vi "experiment control.vi"() -> ()   [LabVIEW 2012] (continued)
            n1914 = Not(x=w4339) -> (.not. x?=w4338:bool)
            n1915 = Bundle By Name(cluster=w4340, "detected"=w4338) -> (w4333:T26)
            n1916 = local write "Trap DDS"(w4333) -> ()
          }
          frame "Trap DDS: IOUpdate" {
            n1917 = local read "Trap DDS"() -> (w4347:T26)
            n1918 = Unbundle By Name(w4347) -> ("detected"=w4348:bool)
            n1919 = case shown="True" w4348 {
              tunnel: w4347 -> [_ w4358]
              tunnel: w4350 -> [w4352 w4355]
              tunnel: [w4352 w4353] -> w4349
              frame False {
              }
              frame True {
                n1920 = Unbundle By Name(w4358) -> ("usb 1"=w4357:refnum<visa-resource-name>, "usb 2"=w4356:refnum<visa-resource-name>)
                n1921 = call "DDS9959 IO Update.vi"("error in (no error)"=w4355, "VISA resource name"=w4357) -> ("error out"=w4354:errorcluster)  [unwired: 4 in, 1 out]
                n1922 = call "DDS9959 IO Update.vi"("error in (no error)"=w4354, "VISA resource name"=w4356) -> ("error out"=w4353:errorcluster)  [unwired: 4 in, 1 out]
              }
            }
          }
          frame "Trap DDS: Upload" {
            n1923 = local read "Trap DDS"() -> (w4360:T26)
            n1924 = Unbundle By Name(w4360) -> ("detected"=w4361:bool)
            n1925 = case shown="True" w4361 {
              tunnel: w4360 -> [_ w4372]
              tunnel: w4363 -> [w4365 w4370]
              tunnel: [w4365 w4371] -> w4362
              frame False {
              }
              frame True {
                n1926 = Unbundle By Name(w4372) -> ("load ARR"=w4369:bool, "ramp enable"=w4368:bool, "channels"=w4373:T95, "Global\nScale Factor"=w4367:dbl, "ramp time"=w4366:u8)
                n1927 = Unbundle By Name(w4372) -> ("usb 1"=w4380:refnum<visa-resource-name>, "clock"=w4382:dbl, "pll multiplier"=w4383:u8, "usb 2"=w4381:refnum<visa-resource-name>)
                n1928 = Array Subset(array=w4373, index=0, length=4) -> (w4378:T95)
                n1929 = Array Subset(array=w4373, index=4, length=4) -> (w4379:T95)
                n1930 = Multiply(x=w4382, y=w4383) -> (x*y=w4384:dbl)
                n1931 = for {
                  tunnel: w4378 -> [w4430] mode=indexing
                  tunnel: w4379 -> [w4429] mode=indexing
                  tunnel: w4380 -> [w4428]
                  tunnel: w4381 -> [w4423]
                  tunnel: w4384 -> [w4420]
                  shift-right: [w4396] -> w4371
                  shift-left: w4370 -> [w4395]
                  tunnel: w4369 -> [w4393]
                  tunnel: w4368 -> [w4392]
                  tunnel: w4366 -> [w4391]
                  tunnel: w4367 -> [w4386]
                  i -> [w4419]
                  w4385 = "04" ("Register")
                  n1932 = Unbundle By Name(w4430) -> ("Frequency"=w4401:dbl, "Phase"=w4422:dbl, "Amplitude"=w4390:dbl)
                  n1933 = Unbundle By Name(w4429) -> ("Frequency"=w4399:dbl, "Phase"=w4421:dbl, "Amplitude"=w4388:dbl)
                  n1934 = Increment(x=w4419) -> (x+1=w4414:i32)
                  n1935 = expression code="x/1000"(w4401) -> (w4400:dbl)
                  n1936 = expression code="x/1000"(w4399) -> (w4398:dbl)
                  n1937 = Bundle By Name(cluster=T48 {"load ARR at ioupdate"=FALSE, "ramp enable"=FALSE, "amplitude multiplier enable"=FALSE, "open"=FALSE, "inc/dec step size (14)"=FALSE, "inc/dec step size (15)"=FALSE} ("Amplitude Control Register"), "load ARR at ioupdate"=w4393, "ramp enable"=w4392, "amplitude multiplier enable"=TRUE) -> (w4413:T48)
                  n1938 = call "DDS9959 Set Frequency.vi"("VISA resource name"=w4428, "Register"=w4385, "Set Frequency (MHz)"=w4400, "Channel"=w4414, "Clock Frequency (MHz)"=w4420, "error in (no error)"=w4395) -> ("VISA resource name out"=w4427:refnum<visa-resource-name>, "error out"=w4404:errorcluster)  [unwired: 8 in]
                  n1939 = call "DDS9959 Set Phase.vi"("VISA resource name"=w4427, "Set Phase (Deg)"=w4422, "Channel"=w4414, "error in (no error)"=w4404) -> ("VISA resource name out"=w4426:refnum<visa-resource-name>, "error out"=w4405:errorcluster)  [unwired: 10 in]
                  n1940 = Multiply(x=w4386, y=w4390) -> (x*y=w4389:dbl)
                  n1941 = Multiply(x=w4386, y=w4388) -> (x*y=w4387:dbl)
                  n1942 = call "DDS9959 Set Amplitude.vi"("VISA resource name"=w4426, "ramp rate"=w4391, "Set Amplitude Scale Factor"=w4389, "Channel"=w4414, "Amplitude Control Register"=w4413, "error in (no error)"=w4405) -> ("VISA resource name out"=w4417:refnum<visa-resource-name>, "error out"=w4418:errorcluster)  [unwired: 8 in]
                  n1943 = Bundle By Name(cluster=T49 {"0=cos, 1=sin"=FALSE, "clear phase accum"=FALSE, "autoclear phase accum"=FALSE, "clear sweep accum"=FALSE, "autoclear sweep accum"=FALSE, "match pipe delays"=FALSE, "DAC power down"=FALSE, "digital power down"=FALSE, "DAC current (8)"=FALSE, "DAC current (9)"=FALSE, "Must be 0"=FALSE, "Open"=FALSE, "Open"=FALSE, "Sweep ramp rate timer"=FALSE, "Sweep enable"=FALSE, "Sweep no-dwell"=FALSE, "Open"=FALSE, "Open"=FALSE, "Open"=FALSE, "Open"=FALSE, "Open"=FALSE, "Open 2"=FALSE, "AFP mod select (22)"=FALSE, "AFP mod select (23)"=FALSE} ("Channel Function Register"), "clear phase accum"=FALSE, "autoclear phase accum"=FALSE, "DAC current (8)"=TRUE, "DAC current (9)"=TRUE) -> (w4407:T49)
                  n1944 = call "DDS9959 Set CFR.vi"("error in (no error)"=w4418, "Channel"=w4414, "Channel Function Register"=w4407, "VISA resource name"=w4417) -> ("error out"=w4397:errorcluster)  [unwired: 1 out]
                  n1945 = call "DDS9959 Set Frequency.vi"("VISA resource name"=w4423, "Register"=w4385, "Set Frequency (MHz)"=w4398, "Channel"=w4414, "Clock Frequency (MHz)"=w4420, "error in (no error)"=w4397) -> ("VISA resource name out"=w4425:refnum<visa-resource-name>, "error out"=w4403:errorcluster)  [unwired: 8 in]
                  n1946 = call "DDS9959 Set Phase.vi"("VISA resource name"=w4425, "Set Phase (Deg)"=w4421, "Channel"=w4414, "error in (no error)"=w4403) -> ("VISA resource name out"=w4424:refnum<visa-resource-name>, "error out"=w4402:errorcluster)  [unwired: 10 in]
                  n1947 = call "DDS9959 Set Amplitude.vi"("VISA resource name"=w4424, "ramp rate"=w4391, "Set Amplitude Scale Factor"=w4387, "Channel"=w4414, "Amplitude Control Register"=w4413, "error in (no error)"=w4402) -> ("VISA resource name out"=w4416:refnum<visa-resource-name>, "error out"=w4415:errorcluster)  [unwired: 8 in]
                  n1948 = call "DDS9959 Set CFR.vi"("error in (no error)"=w4415, "Channel"=w4414, "Channel Function Register"=w4407, "VISA resource name"=w4416) -> ("error out"=w4396:errorcluster)  [unwired: 1 out]
                }
              }
            }
          }
          frame "Trap DDS: Upload Ramp" {
            n1949 = local read "Trap DDS"() -> (w4433:T26)
            n1950 = Unbundle By Name(w4433) -> ("ramp"=w4432:T113, "232"=w4431:refnum<visa-resource-name>)
            n1951 = for {
              tunnel: w4432 -> [w4486] mode=indexing
              shift-right: [w4439] -> w4435
              shift-left: w4436 -> [w4464]
              shift-right: [w4440] -> _
              shift-left: w4431 -> [w4463]
              i -> [w4455]
              w4450 = i16 0 ("lower limit")
              w4449 = i16 1023 ("upper limit")
              w4444 = "w" ("string")
              n1952 = Unbundle By Name(w4486) -> ("start"=w4485:dbl, "end"=w4484:dbl, "ramp time"=w4472:u8, "edge"=w4442:bool)
              n1953 = expression code="x*1024"(w4485) -> (w4483:dbl)
              n1954 = expression code="x*1024"(w4484) -> (w4482:dbl)
              n1955 = Number To Decimal String(number=w4455) -> (decimal integer string=w4443:string)  [unwired: 1 in]
              n1956 = To Word Integer(number=w4483) -> (16bit integer=w4459:i16)
              n1957 = To Word Integer(number=w4482) -> (16bit integer=w4456:i16)
              n1958 = Subtract(x=w4459, y=w4456) -> (x-y=w4479:i16)
              n1959 = Absolute Value(x=w4479) -> (abs(x)=w4478:i16)
              n1960 = Divide(x=w4478, y=i16 1024) -> (x/y=w4476:dbl)
              n1961 = Divide(x=u8 185, y=w4472) -> (x/y=w4470:dbl)
              n1962 = Multiply(x=w4476, y=w4470) -> (x*y=w4475:dbl)
              n1963 = To Unsigned Byte Integer(number=w4475) -> (unsigned 8bit integer=w4454:u8)
              n1964 = case shown="True" w4442 {
                tunnel: ["r" "f"] -> w4441
                frame True {
                }
                frame False {
                }
              }
              n1965 = In Range and Coerce(upper limit=w4449, x=w4459, lower limit=w4450) -> (coerced(x)=w4458:i16)  [unwired: 1 out]
              n1966 = In Range and Coerce(upper limit=w4449, x=w4456, lower limit=w4450) -> (coerced(x)=w4457:i16)  [unwired: 1 out]
              n1967 = In Range and Coerce(upper limit=u8 255, x=w4454, lower limit=u8 1) -> (coerced(x)=w4453:u8)  [unwired: 1 out]
              n1968 = Type Cast(x=w4458) -> (*(type *) &x=w4481:string)  [unwired: 1 in]
              n1969 = Type Cast(x=w4457) -> (*(type *) &x=w4480:string)  [unwired: 1 in]
              n1970 = Type Cast(x=w4453) -> (*(type *) &x=w4474:string)  [unwired: 1 in]
              n1971 = Concatenate Strings(w4444, w4443, "b" ("string"), w4481) -> (w4462:string)
              n1972 = Concatenate Strings(w4444, w4443, "e" ("string"), w4480) -> (w4467:string)
              n1973 = Concatenate Strings(w4444, w4443, "s" ("string"), w4474) -> (w4446:string)
              n1974 = Concatenate Strings(w4444, w4443, w4441) -> (w4445:string)
              n1975 = VISA Write(VISA resource name=w4463, write buffer=w4462, error in (no error)=w4464) -> (VISA resource name out=w4468:refnum<visa-resource-name>, error out=w4469:errorcluster)  [unwired: 1 out]
              n1976 = VISA Write(VISA resource name=w4468, write buffer=w4467, error in (no error)=w4469) -> (VISA resource name out=w4465:refnum<visa-resource-name>, error out=w4466:errorcluster)  [unwired: 1 out]
              n1977 = VISA Write(VISA resource name=w4465, write buffer=w4446, error in (no error)=w4466) -> (VISA resource name out=w4448:refnum<visa-resource-name>, error out=w4447:errorcluster)  [unwired: 1 out]
              n1978 = Wait (ms)(milliseconds to wait=u32 50) -> ()  [unwired: 1 out]
              n1979 = VISA Write(VISA resource name=w4448, write buffer=w4445, error in (no error)=w4447) -> (VISA resource name out=w4440:refnum<visa-resource-name>, error out=w4439:errorcluster)  [unwired: 1 out]
            }
          }
          frame "Trap DDS: Connect Serial" {
            n1980 = local read "Trap DDS"() -> (w4490:T26)
            n1981 = Unbundle By Name(w4490) -> ("232"=w4489:refnum<visa-resource-name>)
            n1982 = call-poly "VISA Configure Serial Port"("VISA resource name"=w4489, "Enable Termination\nChar (T)"=FALSE ("Enable Termination\nChar (T)"), "error in (no error)"=w4494) -> ("error out"=w4493:errorcluster)  [unwired: 11 in, 1 out]
          }
          frame "Trap DDS: Disconnect Serial" {
            n1983 = local read "Trap DDS"() -> (w4497:T26)
            n1984 = Unbundle By Name(w4497) -> ("232"=w4496:refnum<visa-resource-name>)
            n1985 = VISA Close(VISA resource name=w4496, error in (no error)=w4500) -> (error out=w4499:errorcluster)
          }
          frame "Trap DDS: Zero" {
            n1986 = local read "Trap DDS"() -> (w4504:T26)
            n1987 = Unbundle By Name(w4504) -> ("detected"=w4505:bool)
            n1988 = case shown="True" w4505 {
              tunnel: w4504 -> [_ w4514]
              tunnel: w4507 -> [w4509 w4512]
              tunnel: [w4509 w4513] -> w4506
              tunnel: [_ "Trap DDS: IOUpdate" ("State(s) in (\"\")")] -> w4502
              frame False {
              }
              frame True {
                n1989 = Unbundle By Name(w4514) -> ("usb 1"=w4515:refnum<visa-resource-name>, "usb 2"=w4516:refnum<visa-resource-name>)
                n1990 = for {
                  N: 4 -> [_]
                  tunnel: w4515 -> [w4520]
                  tunnel: w4516 -> [w4518]
                  shift-right: [w4521] -> w4513
                  shift-left: w4512 -> [w4519]
                  i -> [w4527]
                  n1991 = Increment(x=w4527) -> (x+1=w4526:i32)
                  n1992 = Bundle By Name(cluster=T49 {"0=cos, 1=sin"=FALSE, "clear phase accum"=FALSE, "autoclear phase accum"=FALSE, "clear sweep accum"=FALSE, "autoclear sweep accum"=FALSE, "match pipe delays"=FALSE, "DAC power down"=FALSE, "digital power down"=FALSE, "DAC current (8)"=FALSE, "DAC current (9)"=FALSE, "Must be 0"=FALSE, "Open"=FALSE, "Open"=FALSE, "Sweep ramp rate timer"=FALSE, "Sweep enable"=FALSE, "Sweep no-dwell"=FALSE, "Open"=FALSE, "Open"=FALSE, "Open"=FALSE, "Open"=FALSE, "Open"=FALSE, "Open 2"=FALSE, "AFP mod select (22)"=FALSE, "AFP mod select (23)"=FALSE} ("Channel Function Register"), "clear phase accum"=TRUE, "autoclear phase accum"=FALSE) -> (w4523:T49)
                  n1993 = call "DDS9959 Set CFR.vi"("error in (no error)"=w4519, "Channel"=w4526, "Channel Function Register"=w4523, "VISA resource name"=w4520) -> ("error out"=w4517:errorcluster)  [unwired: 1 out]
                  n1994 = call "DDS9959 Set CFR.vi"("error in (no error)"=w4517, "Channel"=w4526, "Channel Function Register"=w4523, "VISA resource name"=w4518) -> ("error out"=w4521:errorcluster)  [unwired: 1 out]
                }
              }
            }
            n1995 = Enqueue Element At Opposite End(queue=w4503, element=w4502) -> ()  [unwired: 2 in, 3 out]
          }
          frame "Trap DDS: Reset" {
            n1996 = local read "Trap DDS"() -> (w4528:T26)
            n1997 = Unbundle By Name(w4528) -> ("detected"=w4529:bool)
            n1998 = case shown="True" w4529 {
              tunnel: w4528 -> [_ w4553]
              tunnel: w4532 -> [w4534 w4541]
              tunnel: [w4534 w4539] -> w4531
              frame False {
              }
              frame True {
                w4549 = T104 {"system clock offset"=FALSE, "system clock offset"=FALSE, "open"=FALSE, "open"=FALSE, "multidevice sync mask"=FALSE, "multidevice sync status"=FALSE, "sync master enable"=FALSE, "auto sync enable"=FALSE, "open"=FALSE, "open"=FALSE, "open"=FALSE, "open"=FALSE, "all channel clear phase accumulator"=FALSE, "all channel autoclear phase accumulator"=FALSE, "all channel clear sweep accumulator"=FALSE, "all channel autoclear sweep accumulator"=FALSE} ("Channel Function Register")
                n1999 = Unbundle By Name(w4553) -> ("usb 1"=w4552:refnum<visa-resource-name>, "usb 2"=w4542:refnum<visa-resource-name>)
                n2000 = Bundle By Name(cluster=w4549, "all channel clear phase accumulator"=TRUE) -> (w4547:T104)
                n2001 = call "DDS9959 Set FR2.vi"("error in (no error)"=w4541, "Channel Function Register"=w4547, "VISA resource name"=w4552) -> ("error out"=w4540:errorcluster, "VISA resource name out"=w4546:refnum<visa-resource-name>)  [unwired: 3 in]
                n2002 = Bundle By Name(cluster=w4549, "all channel clear phase accumulator"=FALSE) -> (w4548:T104)
                n2003 = call "DDS9959 IO Update.vi"("error in (no error)"=w4540, "VISA resource name"=w4546) -> ("error out"=w4536:errorcluster, "VISA resource name out"=w4545:refnum<visa-resource-name>)  [unwired: 4 in]
                n2004 = call "DDS9959 Set FR2.vi"("error in (no error)"=w4536, "Channel Function Register"=w4548, "VISA resource name"=w4545) -> ("error out"=w4535:errorcluster)  [unwired: 3 in, 1 out]
                n2005 = call "DDS9959 Set FR2.vi"("error in (no error)"=w4535, "Channel Function Register"=w4547, "VISA resource name"=w4542) -> ("error out"=w4537:errorcluster, "VISA resource name out"=w4544:refnum<visa-resource-name>)  [unwired: 3 in]
                n2006 = call "DDS9959 IO Update.vi"("error in (no error)"=w4537, "VISA resource name"=w4544) -> ("error out"=w4538:errorcluster, "VISA resource name out"=w4543:refnum<visa-resource-name>)  [unwired: 4 in]
                n2007 = call "DDS9959 Set FR2.vi"("error in (no error)"=w4538, "Channel Function Register"=w4548, "VISA resource name"=w4543) -> ("error out"=w4539:errorcluster)  [unwired: 3 in, 1 out]
              }
            }
          }
          frame "---------- Trap DDS ----------" {
            # "Template Separator\n(You can make a copy of, or modify, this frame)"
          }
          frame "DDS: Set Clock" {
            n2008 = local read "DDS"() -> (w4560:T25)
            n2009 = Unbundle By Name(w4560) -> ("address"=w4564:refnum<visa-resource-name>, "pll multiplier"=w4563:u8, "vco gain"=w4559:bool)
            n2010 = call "DDS9959 Set Clock.vi"("error in (no error)"=w4567, "VCO Gain"=w4559, "PLL Multiplier"=w4563, "VISA resource name"=w4564) -> ("error out"=w4566:errorcluster, "VISA resource name out"=w4561:refnum<visa-resource-name>)  [unwired: 6 in]
            n2011 = Unbundle By Name(w4566) -> ("status"=w4558:bool)
            n2012 = Not(x=w4558) -> (.not. x?=w4557:bool)
            n2013 = Bundle By Name(cluster=w4560, "address"=w4561, "detected"=w4557) -> (w4562:T25)
            n2014 = local write "DDS"(w4562) -> ()
          }
          frame "DDS: Set Frequency Ramp" {
            n2015 = local read "DDS"() -> (w4569:T25)
            n2016 = Unbundle By Name(w4569) -> ("address"=w4573:refnum<visa-resource-name>, "frequency ramp"=w4574:bool, "clock"=w4572:dbl)
            n2017 = case shown="True" w4574 {
              tunnel: w4573 -> [w4579 w4589]
              tunnel: [w4580 w4587] -> w4577
              tunnel: w4576 -> [w4580 w4585]
              tunnel: w4572 -> [_ w4583]
              tunnel: [w4579 w4581] -> w4571
              frame False {
              }
              frame True {
                w4582 = 0.002  # Set Frequency (MHz)
                w4584 = u16 2 ("Channel")
                w4594 = 0.5  # Falling Ramp Step (us)
                n2018 = Bundle By Name(cluster=T49 {"0=cos, 1=sin"=FALSE, "clear phase accum"=FALSE, "autoclear phase accum"=FALSE, "clear sweep accum"=FALSE, "autoclear sweep accum"=FALSE, "match pipe delays"=FALSE, "DAC power down"=FALSE, "digital power down"=FALSE, "DAC current (8)"=TRUE, "DAC current (9)"=TRUE, "Must be 0"=FALSE, "Open"=FALSE, "Open"=FALSE, "Sweep ramp rate timer"=FALSE, "Sweep enable"=FALSE, "Sweep no-dwell"=FALSE, "Open"=FALSE, "Open"=FALSE, "Open"=FALSE, "Open"=FALSE, "Open"=FALSE, "Open 2"=FALSE, "AFP mod select (22)"=FALSE, "AFP mod select (23)"=FALSE} ("Channel Function Register"), "Sweep enable"=TRUE, "Sweep no-dwell"=FALSE, "AFP mod select (22)"=FALSE, "AFP mod select (23)"=TRUE) -> (w4601:T49)
                n2019 = call "DDS9959 Set CFR.vi"("error in (no error)"=w4585, "Channel"=w4584, "Channel Function Register"=w4601, "VISA resource name"=w4589) -> ("error out"=w4590:errorcluster, "VISA resource name out"=w4591:refnum<visa-resource-name>)
                n2020 = call "DDS9959 Set Frequency.vi"("VISA resource name"=w4591, "Register"="08", "Set Frequency (MHz)"=w4582, "Channel"=w4584, "Clock Frequency (MHz)"=w4583, "error in (no error)"=w4590) -> ("VISA resource name out"=w4592:refnum<visa-resource-name>, "error out"=w4586:errorcluster)  [unwired: 8 in]
                n2021 = call "DDS9959 Set Frequency.vi"("VISA resource name"=w4592, "Register"="08", "Set Frequency (MHz)"=w4582, "Channel"=w4584, "Clock Frequency (MHz)"=w4583, "error in (no error)"=w4586) -> ("VISA resource name out"=w4593:refnum<visa-resource-name>, "error out"=w4588:errorcluster)  [unwired: 8 in]
                n2022 = call "DDS9959 Set Ramp Rate.vi"("VISA resource name"=w4593, "Falling Ramp Step (us)"=w4594, "Rising Ramp Step (us)"=w4594, "Channel"=w4584, "error in (no error)"=w4588, "Clock Frequency (MHz)"=w4583) -> ("VISA resource name out"=w4581:refnum<visa-resource-name>, "error out"=w4587:errorcluster)  [unwired: 8 in]
              }
            }
            n2023 = Bundle By Name(cluster=w4569, "address"=w4571) -> (w4570:T25)
            n2024 = local write "DDS"(w4570) -> ()
          }
          frame "DDS: Set Frequency" {
            n2025 = local read "DDS"() -> (w4612:T25)
            n2026 = case shown="\"1\", Default" w4618 {
              tunnel: w4612 -> [w4630 w4641 w4652 w4663]
              tunnel: [w4629 w4640 w4651 w4662] -> w4614
              tunnel: [w4624 w4635 w4646 w4657] -> w4605
              tunnel: [w4622 w4633 w4644 w4655] -> w4606
              tunnel: [u16 1 ("Channel") u16 2 ("Channel") u16 3 ("Channel") u16 4 ("Channel")] -> w4604
              tunnel: [w4620 w4631 w4642 w4653] -> w4603
              frame "1", Default {
                n2027 = Unbundle By Name(w4630) -> ("address"=w4629:refnum<visa-resource-name>, "channel 1"=w4623:dbl, "clock"=w4627:dbl, "pll multiplier"=w4626:u8, "channel 1 endramp"=w4621:dbl)
                n2028 = Multiply(x=w4627, y=w4626) -> (x*y=w4625:dbl)
                n2029 = To Double Precision Float(number=w4625) -> (double precision float=w4624:dbl)
                n2030 = expression code="x/2"(w4623) -> (w4622:dbl)
                n2031 = expression code="x/2"(w4621) -> (w4620:dbl)
              }
              frame "2" {
                n2032 = Unbundle By Name(w4641) -> ("address"=w4640:refnum<visa-resource-name>, "channel 2"=w4634:dbl, "clock"=w4638:dbl, "pll multiplier"=w4637:u8, "channel 2 endramp"=w4632:dbl)
                n2033 = Multiply(x=w4638, y=w4637) -> (x*y=w4636:dbl)
                n2034 = To Double Precision Float(number=w4636) -> (double precision float=w4635:dbl)
                n2035 = expression code="x/2"(w4634) -> (w4633:dbl)
                n2036 = expression code="x/2"(w4632) -> (w4631:dbl)
              }
              frame "3" {
                n2037 = Unbundle By Name(w4652) -> ("address"=w4651:refnum<visa-resource-name>, "channel 3"=w4645:dbl, "clock"=w4649:dbl, "pll multiplier"=w4648:u8, "channel 3 endramp"=w4643:dbl)
                n2038 = Multiply(x=w4649, y=w4648) -> (x*y=w4647:dbl)
                n2039 = To Double Precision Float(number=w4647) -> (double precision float=w4646:dbl)
                n2040 = expression code="x/2"(w4645) -> (w4644:dbl)
                n2041 = expression code="x/2"(w4643) -> (w4642:dbl)
              }
              frame "4" {
                n2042 = Unbundle By Name(w4663) -> ("address"=w4662:refnum<visa-resource-name>, "channel 4"=w4656:dbl, "clock"=w4660:dbl, "pll multiplier"=w4659:u8, "channel 4 endramp"=w4654:dbl)
                n2043 = Multiply(x=w4660, y=w4659) -> (x*y=w4658:dbl)
                n2044 = To Double Precision Float(number=w4658) -> (double precision float=w4657:dbl)
                n2045 = expression code="x/2"(w4656) -> (w4655:dbl)
                n2046 = expression code="x/2"(w4654) -> (w4653:dbl)
              }
            }
            n2047 = call "DDS9959 Set Frequency.vi"("VISA resource name"=w4614, "Register"="04", "Set Frequency (MHz)"=w4606, "Channel"=w4604, "Clock Frequency (MHz)"=w4605, "error in (no error)"=w4617) -> ("VISA resource name out"=w4610:refnum<visa-resource-name>, "error out"=w4608:errorcluster)  [unwired: 8 in]
            n2048 = call "DDS9959 Set Frequency.vi"("VISA resource name"=w4610, "Register"="0A", "Set Frequency (MHz)"=w4603, "Channel"=w4604, "Clock Frequency (MHz)"=w4605, "error in (no error)"=w4608) -> ("VISA resource name out"=w4609:refnum<visa-resource-name>, "error out"=w4616:errorcluster)  [unwired: 8 in]
            n2049 = Bundle By Name(cluster=w4612, "address"=w4609) -> (w4613:T25)
            n2050 = local write "DDS"(w4613) -> ()
          }
          frame "DDS: Goto Frequency" {
            n2051 = Match Pattern(string=w4684, regular expression=",") -> (before substring=w4667:string, after substring=w4676:string)  [unwired: 1 in, 2 out]
            n2052 = local read "DDS"() -> (w4669:T25)
            n2053 = case shown="\"1\", Default" w4667 {
              tunnel: w4669 -> [w4730 w4738 w4746 w4754]
              tunnel: [w4729 w4737 w4745 w4753] -> w4681
              tunnel: [w4723 w4731 w4739 w4747] -> w4680
              tunnel: [w4728 w4736 w4744 w4752] -> w4678
              tunnel: [u16 1 ("Channel") u16 2 ("Channel") u16 3 ("Channel") u16 4 ("Channel")] -> w4679
              frame "1", Default {
                n2054 = Unbundle By Name(w4730) -> ("address"=w4729:refnum<visa-resource-name>, "channel 1"=w4728:dbl, "clock"=w4726:dbl, "pll multiplier"=w4725:u8)
                n2055 = Multiply(x=w4726, y=w4725) -> (x*y=w4724:dbl)
                n2056 = To Double Precision Float(number=w4724) -> (double precision float=w4723:dbl)
              }
              frame "2" {
                n2057 = Unbundle By Name(w4738) -> ("address"=w4737:refnum<visa-resource-name>, "channel 2"=w4736:dbl, "clock"=w4734:dbl, "pll multiplier"=w4733:u8)
                n2058 = Multiply(x=w4734, y=w4733) -> (x*y=w4732:dbl)
                n2059 = To Double Precision Float(number=w4732) -> (double precision float=w4731:dbl)
              }
              frame "3" {
                n2060 = Unbundle By Name(w4746) -> ("address"=w4745:refnum<visa-resource-name>, "channel 3"=w4744:dbl, "clock"=w4742:dbl, "pll multiplier"=w4741:u8)
                n2061 = Multiply(x=w4742, y=w4741) -> (x*y=w4740:dbl)
                n2062 = To Double Precision Float(number=w4740) -> (double precision float=w4739:dbl)
              }
              frame "4" {
                n2063 = Unbundle By Name(w4754) -> ("address"=w4753:refnum<visa-resource-name>, "channel 4"=w4752:dbl, "clock"=w4750:dbl, "pll multiplier"=w4749:u8)
                n2064 = Multiply(x=w4750, y=w4749) -> (x*y=w4748:dbl)
                n2065 = To Double Precision Float(number=w4748) -> (double precision float=w4747:dbl)
              }
            }
            n2066 = Fract/Exp String To Number(string=w4676) -> (number=w4672:dbl)  [unwired: 3 in, 1 out]
            n2067 = expression code="x/2"(w4672) -> (w4671:dbl)
            n2068 = expression code="x/2"(w4678) -> (w4673:dbl)
            n2069 = Subtract(x=w4671, y=w4673) -> (x-y=w4675:dbl)
            n2070 = Sign(1:w4675) -> (0:w4674:dbl)
            n2071 = while {
              tunnel: w4680 -> [w4720]
              tunnel: w4679 -> [w4719]
              shift-right: [w4704] -> w4666
              shift-left: w4673 -> [w4705]
              shift-right: [w4706] -> w4682
              shift-left: w4683 -> [w4722]
              tunnel: w4674 -> [w4716]
              tunnel: w4671 -> [w4711]
              tunnel: w4673 -> [w4712]
              shift-right: [w4708] -> w4668
              shift-left: w4681 -> [w4721]
              stop <- w4710 stop-if-true
              n2072 = Multiply(x=w4716, y=0.5) -> (x*y=w4718:dbl)
              n2073 = Wait (ms)(milliseconds to wait=u32 10) -> ()  [unwired: 1 out]
              n2074 = Add(x=w4705, y=w4718) -> (x+y=w4715:dbl)
              n2075 = Max & Min(x=w4712, y=w4711) -> (max(x,y)=w4714:dbl, min(x,y)=w4713:dbl)
              n2076 = In Range and Coerce(upper limit=w4714, x=w4715, lower limit=w4713) -> (coerced(x)=w4704:dbl)  [unwired: 1 out]
              n2077 = Equal?(x=w4704, y=w4711) -> (x = y?=w4710:bool)
              n2078 = call "DDS9959 Set Frequency.vi"("VISA resource name"=w4721, "Register"="04", "Set Frequency (MHz)"=w4704, "Channel"=w4719, "Clock Frequency (MHz)"=w4720, "error in (no error)"=w4722) -> ("VISA resource name out"=w4709:refnum<visa-resource-name>, "error out"=w4707:errorcluster)  [unwired: 8 in]
              n2079 = call "DDS9959 IO Update.vi"("error in (no error)"=w4707, "VISA resource name"=w4709) -> ("error out"=w4706:errorcluster, "VISA resource name out"=w4708:refnum<visa-resource-name>)  [unwired: 4 in]
            }
            n2080 = expression code="2*x"(w4666) -> (w4665:dbl)
            n2081 = case shown="\"1\", Default" w4667 {
              tunnel: [w4689 w4693 w4697 w4701] -> w4670
              tunnel: w4669 -> [w4688 w4692 w4696 w4700]
              tunnel: w4668 -> [w4687 w4691 w4695 w4699]
              tunnel: w4665 -> [w4686 w4690 w4694 w4698]
              frame "1", Default {
                n2082 = Bundle By Name(cluster=w4688, "address"=w4687, "channel 1"=w4686) -> (w4689:T25)
              }
              frame "2" {
                n2083 = Bundle By Name(cluster=w4692, "address"=w4691, "channel 2"=w4690) -> (w4693:T25)
              }
              frame "3" {
                n2084 = Bundle By Name(cluster=w4696, "address"=w4695, "channel 3"=w4694) -> (w4697:T25)
              }
              frame "4" {
                n2085 = Bundle By Name(cluster=w4700, "address"=w4699, "channel 4"=w4698) -> (w4701:T25)
              }
            }
            n2086 = local write "DDS"(w4670) -> ()
          }
          frame "---------- Coils ----------" {
            # "Template Separator\n(You can make a copy of, or modify, this frame)"
          }
          frame "Coils: Initialize" {
            # "Template Separator\n(You can make a copy of, or modify, this frame)"
            n2087 = local read "Coils"() -> (w4762:T15)
            n2088 = Unbundle By Name(w4762) -> ("Keithley USB"=w4768:refnum<visa-resource-name>, "AO Channels"=w4767:tag, "DO Lines"=w4766:tag)
            n2089 = call "CoilsInit.vi"("error in"=w4765, "DO Lines"=w4766, "AO Channels"=w4767, "Keithley USB"=w4768) -> ("error out"=w4759:errorcluster, "DO Task out"=w4763:refnum<k21>, "AO Task out"=w4764:refnum<k21>)  [unwired: 4 in, 1 out]
            n2090 = local write "Coils AO Task:skip"(w4764) -> ()
            n2091 = local write "Coils DO Task:skip"(w4763) -> ()
            n2092 = Unbundle By Name(w4759) -> ("status"=w4758:bool)
            n2093 = case shown="False" w4758 {
              tunnel: w4761 -> [w4772 w4773]
              tunnel: [w4771 w4773] -> w4760
              frame False {
                n2094 = Enqueue Element At Opposite End(queue=w4772, element="Coils: Set") -> (queue out=w4771:refnum<queue>)  [unwired: 2 in, 2 out]
              }
              frame True {
              }
            }
          }
          frame "Coils: Close" {
            # "Template Separator\n(You can make a copy of, or modify, this frame)"
            n2095 = local read "Coils AO Task:skip"() -> (w4775:refnum<k21>)
            n2096 = local read "Coils DO Task:skip"() -> (w4774:refnum<k21>)
            n2097 = local read "Coils"() -> (w4780:T15)
            n2098 = Unbundle By Name(w4780) -> ("Keithley USB"=w4778:refnum<visa-resource-name>)
            n2099 = call "CoilsClose.vi"("error in"=w4777, "Coils DO Task in"=w4774, "Coils AO Task in"=w4775, "Keithley USB"=w4778) -> ("error out"=w4776:errorcluster)  [unwired: 7 in]
          }
          frame "Coils: Set" {
            # "Template Separator\n(You can make a copy of, or modify, this frame)"
            n2100 = flat-sequence {
              tunnel: w4784 -> [w4793]
              tunnel: w4783 -> [w4871]
              tunnel: [w4870] -> w4782
              frame #0 {
                n2101 = Index Array(array=w4793, index=0) -> (element=w4789:string)
                n2102 = Index Array(array=w4793, index=1) -> (element=w4788:string)
                n2103 = Index Array(array=w4793, index=2) -> (element=w4787:string)
                n2104 = case shown="\"\", Default" w4789 {
                  selector: w4789 -> [_ _ _ w4841]
                  tunnel: w4788 -> [w4796 w4811 w4826 w4839]
                  tunnel: w4787 -> [w4795 w4810 w4825 _]
                  frame "Magnetometer Shim" {
                    n2105 = Fract/Exp String To Number(string=w4795) -> (number=w4794:dbl)  [unwired: 3 in, 1 out]
                    n2106 = case shown="\"\", Default" w4796 {
                      tunnel: w4794 -> [w4797 w4800 w4803 w4806 _]
                      frame "x" {
                        n2107 = local read "Coils"() -> (w4799:T15)
                        n2108 = Bundle By Name(cluster=w4799, "Magnetometer Shim.x"=w4797) -> (w4798:T15)
                        n2109 = local write "Coils"(w4798) -> ()
                      }
                      frame "y" {
                        n2110 = local read "Coils"() -> (w4802:T15)
                        n2111 = Bundle By Name(cluster=w4802, "Magnetometer Shim.y"=w4800) -> (w4801:T15)
                        n2112 = local write "Coils"(w4801) -> ()
                      }
                      frame "z" {
                        n2113 = local read "Coils"() -> (w4805:T15)
                        n2114 = Bundle By Name(cluster=w4805, "Magnetometer Shim.z"=w4803) -> (w4804:T15)
                        n2115 = local write "Coils"(w4804) -> ()
                      }
                      frame "axgrad" {
                        n2116 = local read "Coils"() -> (w4808:T15)
                        n2117 = Bundle By Name(cluster=w4808, "Magnetometer Shim.axgrad"=w4806) -> (w4807:T15)
                        n2118 = local write "Coils"(w4807) -> ()
                      }
                      frame "", Default {
                      }
                    }
                  }
                  frame "Ion Shim" {
                    n2119 = Fract/Exp String To Number(string=w4810) -> (number=w4809:dbl)  [unwired: 3 in, 1 out]
                    n2120 = case shown="\"x\"" w4811 {
                      tunnel: w4809 -> [w4812 w4815 w4818 w4821 _]
                      frame "x" {
                        n2121 = local read "Coils"() -> (w4814:T15)
                        n2122 = Bundle By Name(cluster=w4814, "Ion Shim.x"=w4812) -> (w4813:T15)
                        n2123 = local write "Coils"(w4813) -> ()
                      }
                      frame "y" {
                        n2124 = local read "Coils"() -> (w4817:T15)
                        n2125 = Bundle By Name(cluster=w4817, "Ion Shim.y"=w4815) -> (w4816:T15)
                        n2126 = local write "Coils"(w4816) -> ()
                      }
                      frame "z" {
                        n2127 = local read "Coils"() -> (w4820:T15)
                        n2128 = Bundle By Name(cluster=w4820, "Ion Shim.z"=w4818) -> (w4819:T15)
                        n2129 = local write "Coils"(w4819) -> ()
                      }
                      frame "axgrad" {
                        n2130 = local read "Coils"() -> (w4823:T15)
                        n2131 = Bundle By Name(cluster=w4823, "Ion Shim.axgrad"=w4821) -> (w4822:T15)
                        n2132 = local write "Coils"(w4822) -> ()
                      }
                      frame "", Default {
                      }
                    }
                  }
                  frame "Bias" {
                    n2133 = Fract/Exp String To Number(string=w4825) -> (number=w4824:dbl)  [unwired: 3 in, 1 out]
                    n2134 = case shown="\"x\"" w4826 {
                      tunnel: w4824 -> [w4827 w4830 w4833 w4836 _]
                      frame "x" {
                        n2135 = local read "Coils"() -> (w4829:T15)
                        n2136 = Bundle By Name(cluster=w4829, "Bias.x"=w4827) -> (w4828:T15)
                        n2137 = local write "Coils"(w4828) -> ()
                      }
                      frame "y" {
                        n2138 = local read "Coils"() -> (w4832:T15)
                        n2139 = Bundle By Name(cluster=w4832, "Bias.y"=w4830) -> (w4831:T15)
                        n2140 = local write "Coils"(w4831) -> ()
                      }
                      frame "z" {
                        n2141 = local read "Coils"() -> (w4835:T15)
                        n2142 = Bundle By Name(cluster=w4835, "Bias.z"=w4833) -> (w4834:T15)
                        n2143 = local write "Coils"(w4834) -> ()
                      }
                      frame "axgrad" {
                        n2144 = local read "Coils"() -> (w4838:T15)
                        n2145 = Bundle By Name(cluster=w4838, "Bias.axgrad"=w4836) -> (w4837:T15)
                        n2146 = local write "Coils"(w4837) -> ()
                      }
                      frame "", Default {
                      }
                    }
                  }
                  frame "", Default {
                    n2147 = Fract/Exp String To Number(string=w4839) -> (number=w4840:dbl)  [unwired: 3 in, 1 out]
                    n2148 = case shown="\"1\"" w4841 {
                      tunnel: w4840 -> [w4842 w4845 w4848 w4851 _ _ _]
                      frame "x" {
                        n2149 = local read "Coils"() -> (w4844:T15)
                        n2150 = Bundle By Name(cluster=w4844, "Bias.x"=w4842) -> (w4843:T15)
                        n2151 = local write "Coils"(w4843) -> ()
                      }
                      frame "y" {
                        n2152 = local read "Coils"() -> (w4847:T15)
                        n2153 = Bundle By Name(cluster=w4847, "Bias.y"=w4845) -> (w4846:T15)
                        n2154 = local write "Coils"(w4846) -> ()
                      }
                      frame "z" {
                        n2155 = local read "Coils"() -> (w4850:T15)
                        n2156 = Bundle By Name(cluster=w4850, "Bias.z"=w4848) -> (w4849:T15)
                        n2157 = local write "Coils"(w4849) -> ()
                      }
                      frame "axgrad" {
                        n2158 = local read "Coils"() -> (w4853:T15)
                        n2159 = Bundle By Name(cluster=w4853, "Bias.axgrad"=w4851) -> (w4852:T15)
                        n2160 = local write "Coils"(w4852) -> ()
                      }
                      frame "0" {
                        n2161 = local read "Coils"() -> (w4856:T15)
                        n2162 = Bundle By Name(cluster=w4856, "Current Toggle"=FALSE) -> (w4855:T15)
                        n2163 = local write "Coils"(w4855) -> ()
                      }
                      frame "1" {
                        n2164 = local read "Coils"() -> (w4859:T15)
                        n2165 = Bundle By Name(cluster=w4859, "Current Toggle"=TRUE) -> (w4858:T15)
                        n2166 = local write "Coils"(w4858) -> ()
                      }
                      frame "", Default {
                      }
                    }
                  }
                }
              }
              frame #1 {
                n2167 = local read "Coils"() -> (w4866:T15)
                n2168 = Unbundle By Name(w4866) -> ("Magnetometer Shim"=w4864:cluster{"x":dbl, "y":dbl, "z":dbl, "axgrad":dbl}, "Ion Shim"=w4863:cluster{"x":dbl, "y":dbl, "z":dbl, "axgrad":dbl}, "Bias"=w4861:cluster{"x":dbl, "y":dbl, "z":dbl, "axgrad":dbl})
                n2169 = Add(x=w4864, y=w4863) -> (x+y=w4862:cluster{"x":dbl, "y":dbl, "z":dbl, "axgrad":dbl})
                n2170 = Add(x=w4862, y=w4861) -> (x+y=w4860:cluster{"x":dbl, "y":dbl, "z":dbl, "axgrad":dbl})
                n2171 = Bundle By Name(cluster=w4866, "Total"=w4860) -> (w4865:T15)
                n2172 = local write "Coils"(w4865) -> ()
              }
              frame #2 {
                n2173 = local read "Coils"() -> (w4872:T15)
                n2174 = local read "Coils AO Task:skip"() -> (w4868:refnum<k21>)
                n2175 = local read "Coils DO Task:skip"() -> (w4867:refnum<k21>)
                n2176 = Unbundle By Name(w4872) -> ("Total"=w4873:cluster{"x":dbl, "y":dbl, "z":dbl, "axgrad":dbl}, "Keithley USB"=w4874:refnum<visa-resource-name>, "Current Toggle"=w4869:bool)
                n2177 = case shown="True" w4869 {
                  tunnel: w4874 -> [w4880 w4886]
                  tunnel: w4873 -> [w4879 _]
                  tunnel: w4871 -> [w4878 w4885]
                  tunnel: [w4877 w4884] -> w4870
                  tunnel: w4868 -> [w4876 w4883]
                  tunnel: w4867 -> [w4875 w4882]
                  frame True {
                    n2178 = call "CoilsSet.vi"("Settings"=w4879, "error in"=w4878, "DO Task"=w4875, "AO Task"=w4876, "Keithley USB"=w4880) -> ("error out"=w4877:errorcluster)  [unwired: 3 in, 3 out]
                  }
                  frame False {
                    n2179 = call "CoilsSet.vi"("Settings"=cluster{"x":dbl, "y":dbl, "z":dbl, "axgrad":dbl} {"x"=0.0, "y"=0.0, "z"=0.0, "axgrad"=0.0}, "error in"=w4885, "DO Task"=w4882, "AO Task"=w4883, "Keithley USB"=w4886) -> ("error out"=w4884:errorcluster)  [unwired: 3 in, 3 out]
                  }
                }
              }
            }
          }
          frame "---------- DAC ----------" {
            # "Template Separator\n(You can make a copy of, or modify, this frame)"
          }
          frame "DAC: Upload2" {
            n2180 = Unbundle By Name(w4891) -> ("dac state.loaded"=w4892:bool)
            n2181 = case shown="False" w4892 {
              tunnel: w4896 -> [w4910 w4956]
              tunnel: w4894 -> [w4925 w4954]
              tunnel: [w4923 w4954] -> w4895
              tunnel: w4893 -> [_ w4953]
              tunnel: w4891 -> [w4900 w4949]
              tunnel: [w4897 w4949] -> w4890
              frame False {
                n2182 = Match Pattern(string=w4910, regular expression=",") -> (before substring=w4906:string, after substring=w4911:string)  [unwired: 1 in, 2 out]
                n2183 = local read "DAC Kick 2"() -> (w4915:T8)
                n2184 = Decimal String To Number(string=w4906) -> (number=w4907:i32)  [unwired: 2 in, 1 out]
                n2185 = for {
                  tunnel: w4915 -> [w4942] mode=indexing
                  tunnel: [w4941] -> w4914 mode=indexing
                  n2186 = Unbundle By Name(w4942) -> ("Name"=w4941:string)
                }
                n2187 = local read "DAC Schedule"() -> (w4908:T6)
                n2188 = local read "DAC Tasks"() -> (w4909:T8)
                n2189 = Search 1D Array(1D array=w4914, element=w4911) -> (index of element=w4919:i32)  [unwired: 1 in]
                n2190 = property on="DAC Kick 2" class="Arr (strict)"() -> ("Index Values"=w4902:u32[])  [unwired: 2 in, 2 out]
                n2191 = call "DAC compile.vi"("DAC Tasks"=w4909, "DAC Schedule"=w4908, "index"=w4907) -> ("DAC"=w4905:cluster{"Time":dbl, "Voltage":dbl[]}[])  [unwired: 8 in]
                n2192 = Index Array(array=w4902) -> (element=w4918:u32)  [unwired: 1 in]
                n2193 = Greater Or Equal To 0?(x=w4919) -> (x >= 0?=w4917:bool)
                n2194 = for {
                  tunnel: w4905 -> [w4948] mode=indexing
                  tunnel: [w4947] -> w4903 mode=indexing
                  tunnel: [w4946] -> w4904 mode=indexing
                  n2195 = Unbundle By Name(w4948) -> ("Time"=w4947:dbl, "Voltage"=w4946:dbl[])
                }
                n2196 = Select(t=w4919, s=w4917, f=w4918) -> (s? t:f=w4920:u32)
                n2197 = Index Array(array=w4915, index=w4920) -> (element=w4916:T55)
                n2198 = Unbundle By Name(w4916) -> ("DAC"=w4913:cluster{"Time":dbl, "Voltage":dbl[]}[])
                n2199 = for {
                  tunnel: w4913 -> [w4945] mode=indexing
                  tunnel: [w4944] -> w4928 mode=indexing
                  tunnel: [w4943] -> w4926 mode=indexing
                  n2200 = Unbundle By Name(w4945) -> ("Time"=w4944:dbl, "Voltage"=w4943:dbl[])
                }
                n2201 = Transpose 2D Array(2D array=w4904) -> (transposed array=w4938:dbl[][])
                n2202 = Transpose 2D Array(2D array=w4926) -> (transposed array=w4929:dbl[][])
                n2203 = Array Subset(array=w4938, index (row)=0 ("index"), length (row)=8 ("length")) -> (w4937:dbl[][])  [unwired: 2 in]
                n2204 = Array Subset(array=w4929, index (row)=0 ("index"), length (row)=6 ("length")) -> (w4930:dbl[][])  [unwired: 2 in]
                n2205 = call "DAC upload.vi"("dt"="DAC Resolution", "error in"=w4925, "voltage"=w4937, "time"=w4903, "device"=tag "DAC_SHIM") -> ("error out"=w4924:errorcluster, "clock"=w4935:refnum<k21>, "output"=w4936:refnum<k21>)  [unwired: 4 in]
                n2206 = call "DAC upload.vi"("dt"="DAC Resolution", "error in"=w4924, "voltage"=w4930, "time"=w4928, "device"=tag "DAC_KICK") -> ("error out"=w4923:errorcluster, "clock"=w4921:refnum<k21>, "output"=w4922:refnum<k21>)  [unwired: 4 in]
                n2207 = Unbundle By Name(w4900) -> ("dac state"=w4898:T7)
                n2208 = Bundle By Name(cluster=w4898, "output 1"=w4936, "clock 1"=w4935, "output 2"=w4922, "clock 2"=w4921, "loaded"=TRUE) -> (w4899:T7)
                n2209 = Bundle By Name(cluster=w4900, "dac state"=w4899) -> (w4897:T52)
              }
              frame True {
                n2210 = Concatenate Strings("DAC: Upload2 >> ", w4956) -> (w4950:string)
                n2211 = Enqueue Element At Opposite End(queue=w4953, element=w4950) -> (queue out=w4952:refnum<queue>)  [unwired: 2 in, 2 out]
                n2212 = Enqueue Element At Opposite End(queue=w4952, element="DAC: Clear") -> ()  [unwired: 2 in, 3 out]
              }
            }
          }
          frame "DAC: View" {
            n2213 = Match Pattern(string=w4969, regular expression=",") -> (before substring=w4963:string)  [unwired: 1 in, 3 out]
